vi "Event Frame Page.vi"(8 "error in (no error)":errorcluster, 11 "Node Ptr":T1 format="%.0x") -> (0 "error out":errorcluster)   [LabVIEW 2015, in "J1939 Addon System Explorer.lvlib"]
uses:
  J1939 Addon System Explorer.lvlib
  <vilib>/NI Veristand/Custom Device API/Custom Device Item Ref.ctl
  Shared/Types/XNET Frame Event Properties.ctl
  Shared/J1939 Utilities/SubVIs/Convert CAN Arb ID to J1939 ID.vi
  Shared/SubVIs/Constants.vi
  <vilib>/NI Veristand/Custom Device API/Get Item Property (U32).vi
  <vilib>/NI Veristand/Custom Device API/Get Item Property (Variant).vi
  <vilib>/NI Veristand/Custom Device API/Set Item Property (Variant).vi
  <vilib>/NI VeriStand/Custom Device API/Custom Device API.lvlib
  Shared/J1939 Addon Shared.lvlib
  Shared/J1939 Utilities/J1939 Utilities.lvlib
panel:
  in  "Description":string
  out "Source Address":u8
  out "Priority":u8
  out "PGN":u32
  in  "SHDocVw.IWebBrowser2":refnum<k7>(container)
  in  "Transimission Trigger":cluster{"Section Name":string}={"Section Name"="Transmission Trigger"}
  out "Frame ID":u32
  in  "Enable software cyclic trigger":bool
  in  "Transmit trigger":enum16{"Channel value change"}(ring)
  in  "Transmit Time":dbl format="%#_p"
  in  "Custom Device Settings":cluster{"Section Name":string}={"Section Name"="Custom Device Item Settings"}
  out "Name":string
  # "secs"
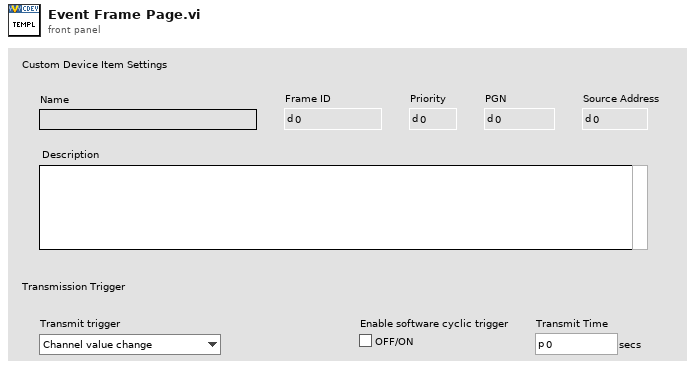
[diagram p1: front panel]
types:
  T1 = typedef "Custom Device API.lvlib/Custom Device Item Ref.ctl" = u64
  T2 = typedef "J1939 Addon Shared.lvlib/XNET Frame Event Properties.ctl" = cluster{"Transmit trigger":enum16{"Channel value change"}, "Enable software cyclic trigger":bool, "Transmit Time":dbl}
  T3 = typedef "Custom Device API.lvlib/Custom Device Item Info.ctl" = cluster{"Name":string, "Is Channel":bool, "GUID":string, "Is Waveform":bool}
  T4 = enum8{"Enabled", "Disabled", "Disabled and Grayed Out"}
  T5 = typedef "Custom Device API.lvlib/Custom Device Commands.ctl" = enum16{"Default", "Item renamed", "Shutdown", "Dynamic button pressed"}
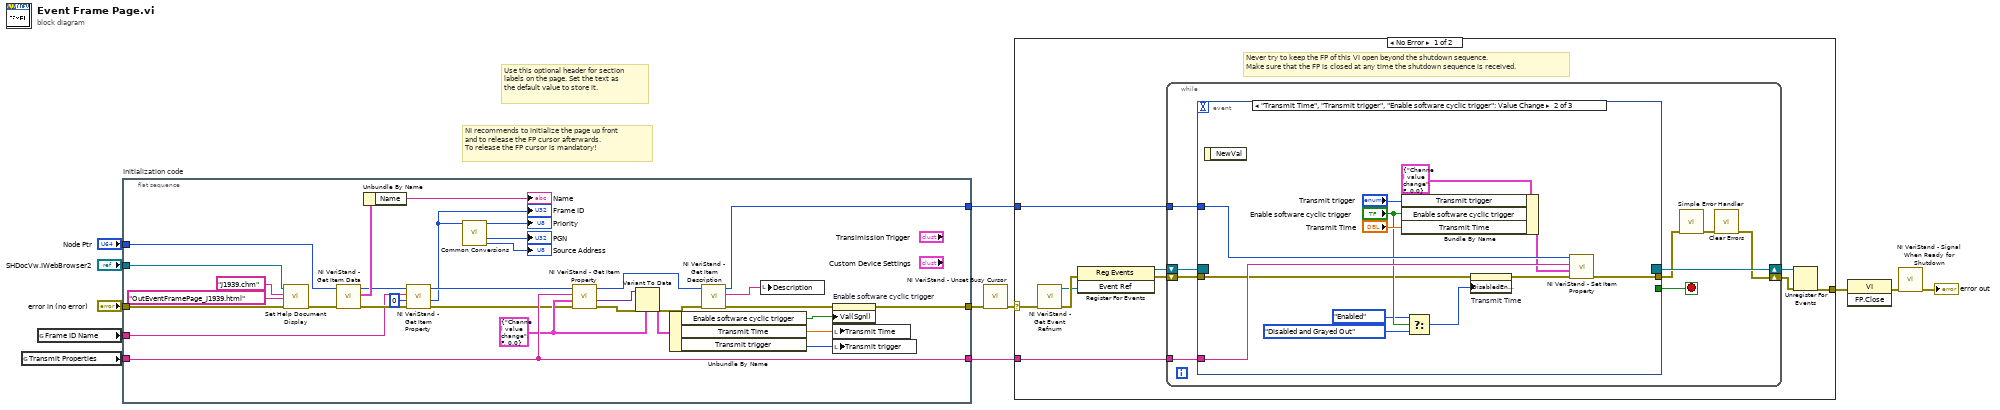
[diagram p0: block diagram]
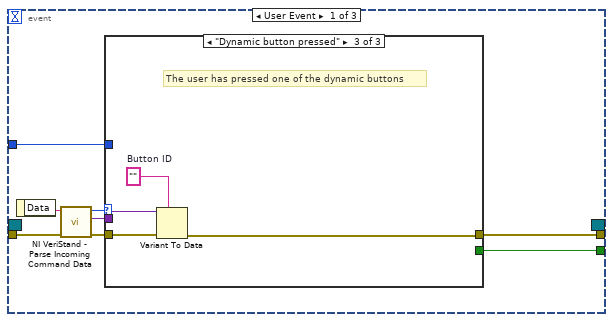
[diagram p2: hidden frame]
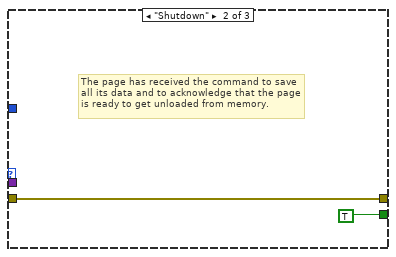
[diagram p4: hidden frame]
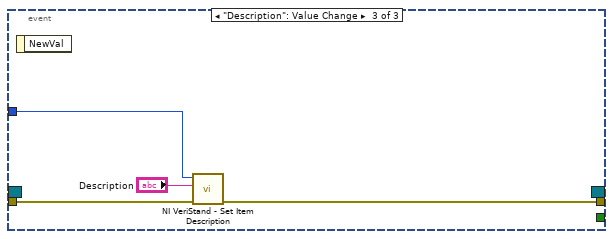
[diagram p5: hidden frame]
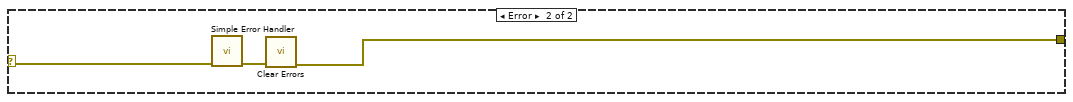
[diagram p6: hidden frame]
diagram:
  # "Use this optional header for section labels on the page. Set the text as the default value to store it."
  # "NI recommends to initialize the page up front\nand to release the FP cursor afterwards.\nTo release the FP cursor is mandatory!"
  n1 = global read "Constants.vi" "Transmit Properties"() -> (w4:string)
  n2 = global read "Constants.vi" "Frame ID Name"() -> (w1:string)
  n3 = flat-sequence "Initialization code" {
    tunnel: "error in (no error)" -> [w39]
    tunnel: "Node Ptr" -> [w42]
    tunnel: [w13] -> w8
    tunnel: [w17] -> w5
    tunnel: w4 -> [w43]
    tunnel: [w43] -> w3
    tunnel: "SHDocVw.IWebBrowser2" -> [w37]
    tunnel: w1 -> [w25]
    frame #0 {
      w34 = T2 {"Transmit trigger"=enum."Channel value change", "Enable software cyclic trigger"=FALSE, "Transmit Time"=0.0} ("Transmit Properties")
      n4 = call "Set Help Document Display.vi"("error in (no error)"=w39, "HTML File"="OutEventFramePage_J1939.html", "Main CHM File"="J1939.chm", "SHDocVw.IWebBrowser2"=w37) -> ("error out"=w38:errorcluster)  [unwired: 7 in]
      n5 = call <vilib>:"NI VeriStand - Get Item Data.vi"("error in (no error)"=w38, "Item Ref in"=w42) -> ("error out"=w30:errorcluster, "Item Info"=w44:T3, "Item Ref out"=w28:T1)  [unwired: 7 out]
      n6 = Unbundle By Name(w44) -> ("Name"=→"Name":string)
      n7 = call-poly <vilib>:"NI VeriStand - Get Item Property.vi"("error in (no error)"=w30, "Default Value"=u32 0, "Property Name"=w25, "Item Ref in"=w28) -> ("error out"=w29:errorcluster, "Value"=w24:u32, "Item Ref out"=w27:T1)  [unwired: 4 in, 1 out]
      "Frame ID" <- w24
      n8 = call-poly "Common Conversions.vi"("Arb ID"=w24) -> ("Priority"=→"Priority":u8, "PGN"=→"PGN":u32, "Source Address"=→"Source Address":u8)  [unwired: 11 in, 1 out]
      n9 = call-poly <vilib>:"NI VeriStand - Get Item Property.vi"("error in (no error)"=w29, "Default Value"=w34, "Property Name"=w43, "Item Ref in"=w27) -> ("error out"=w36:errorcluster, "Value"=w35:variant, "Item Ref out"=w18:T1)  [unwired: 4 in, 1 out]
      n10 = Variant To Data(error in=w36, type=w34, Variant=w35) -> (data=w33:T2, error out=w19:errorcluster)
      n11 = Unbundle By Name(w33) -> ("Enable software cyclic trigger"=w14:bool, "Transmit Time"=w32:dbl, "Transmit trigger"=w31:enum16{"Channel value change"})
      n12 = call <vilib>:"NI VeriStand - Get Item Description.vi"("error in (no error)"=w19, "Item Ref in"=w18) -> ("error out"=w15:errorcluster, "Description"=w16:string, "Item Ref out"=w17:T1)  [unwired: 7 out]
      n13 = local write "Description"(w16) -> ()
      n14 = property on="Enable software cyclic trigger" class="Bool (strict)"(error in=w15, "Val(Sgnl)"=w14) -> (error out=w13:errorcluster)  [unwired: 1 in, 1 out]
      n15 = local write "Transmit Time"(w32) -> ()
      n16 = local write "Transmit trigger"(w31) -> ()
    }
  }
  n17 = call <vilib>:"NI VeriStand - Unset Busy Cursor.vi"("error in (no error)"=w8) -> ("error out"=w7:errorcluster)  [unwired: 10 out]
  n18 = case shown="No Error" w7 {
    selector: w7 -> [w46 w98]
    tunnel: [w51 w96] -> w12
    tunnel: w5 -> [w47 _]
    tunnel: w3 -> [w45 _]
    frame No Error {
      # "Never try to keep the FP of this VI open beyond the shutdown sequence.\nMake sure that the FP is closed at any time the shutdown sequence is received."
      n19 = call <vilib>:"NI VeriStand - Get Event Refnum.vi"("error in (no error)"=w46) -> ("error out"=w54:errorcluster, "Event Ref"=w50:refnum<user-event>)  [unwired: 9 out]
      n20 = register-events(error in=w54, w50) -> (reference out=w48:refnum<event-registration>, error out=w49:errorcluster)  [unwired: 1 in]
      n21 = while {
        tunnel: w47 -> [w59]
        shift-right: [w56] -> w52
        shift-left: w49 -> [w62]
        shift-right: [w63] -> w53
        shift-left: w48 -> [w61]
        tunnel: w45 -> [w55]
        stop <- w60 stop-if-true
        n22 = event shown="[1] \"Transmit Time\", \"Transmit trigger\", \"Enable software cyclic trigger\": Value Change" {
          selector: w61 -> [_ _ _]
          dyn-events: [_ _ _] -> w63
          timeout: _ -> [_ _ _]
          tunnel: w62 -> [w71 w80 w94]
          tunnel: [w67 _ _] -> w60
          tunnel: [w66 w91 w93] -> w58
          tunnel: w59 -> [w65 w90 w92]
          tunnel: w55 -> [_ w89 _]
          event User Event {
            n23 = event-data() -> ("Data"=w70:string)  [unwired: 1 out]
            n24 = call <vilib>:"NI VeriStand - Parse Incoming Command Data.vi"("error in (no error)"=w71, "Incoming data"=w70) -> ("error out"=w69:errorcluster, "Outgoing data"=w64:variant, "Action"=w68:T5)  [unwired: 7 out]
            n25 = case shown="\"Dynamic button pressed\"" w68 {
              tunnel: w69 -> [w72 w73 w78]
              tunnel: [_ TRUE _] -> w67
              tunnel: [w72 w73 w75] -> w66
              tunnel: w65 -> [_ _ _]
              tunnel: w64 -> [_ _ w77]
              frame "Default", Default {
              }
              frame "Shutdown" {
                # "The page has received the command to save all its data and to acknowledge that the page is ready to get unloaded from memory."
              }
              frame "Dynamic button pressed" {
                w76 = ""  # Button ID
                # "The user has pressed one of the dynamic buttons"
                n26 = Variant To Data(error in=w78, type=w76, Variant=w77) -> (error out=w75:errorcluster)  [unwired: 1 out]
              }
            }
          }
          event "Transmit Time", "Transmit trigger", "Enable software cyclic trigger": Value Change {
            n27 = event-data() -> ()  [unwired: 2 out]
            n28 = Bundle By Name(cluster=T2 {"Transmit trigger"=enum."Channel value change", "Enable software cyclic trigger"=FALSE, "Transmit Time"=0.0} ("Transmit Properties"), "Transmit trigger"="Transmit trigger", "Enable software cyclic trigger"="Enable software cyclic trigger", "Transmit Time"="Transmit Time") -> (w85:T2)
            n29 = Select(t=T4."Enabled" ("Disabled"), s="Enable software cyclic trigger", f=T4."Disabled and Grayed Out") -> (s? t:f=w81:T4)
            n30 = property on="Transmit Time" class="DigNum (strict)"(error in=w80, "DisabledEnum"=w81) -> (error out=w79:errorcluster)  [unwired: 1 in, 1 out]
            n31 = call-poly <vilib>:"NI VeriStand - Set Item Property.vi"("error in (no error)"=w79, "Value"=w85, "Property Name"=w89, "Item Ref in"=w90) -> ("error out"=w91:errorcluster)  [unwired: 5 in, 2 out]
          }
          event "Description": Value Change {
            n32 = event-data() -> ()  [unwired: 2 out]
            n33 = call <vilib>:"NI VeriStand - Set Item Description.vi"("error in (no error)"=w94, "Description"="Description", "Item Ref in"=w92) -> ("error out"=w93:errorcluster)  [unwired: 8 out]
          }
        }
        n34 = call <vilib>:"Simple Error Handler.vi"("error in (no error)"=w58) -> ("error out"=w57:errorcluster)  [unwired: 1 in, 7 out]
        n35 = call <vilib>:"Clear Errors.vi"("error in (no error)"=w57) -> ("error out"=w56:errorcluster)  [unwired: 1 in, 5 out]
      }
      n36 = Unregister For Events(event registration refnum=w53, error in=w52) -> (error out=w51:errorcluster)
    }
    frame Error {
      n37 = call <vilib>:"Simple Error Handler.vi"("error in (no error)"=w98) -> ("error out"=w97:errorcluster)  [unwired: 1 in, 7 out]
      n38 = call <vilib>:"Clear Errors.vi"("error in (no error)"=w97) -> ("error out"=w96:errorcluster)  [unwired: 1 in, 5 out]
    }
  }
  n39 = invoke class="VI" method="FP.Close"(error in=w12) -> (error out=w11:errorcluster)  [unwired: 2 in, 2 out]
  n40 = call <vilib>:"NI VeriStand - Signal When Ready for Shutdown.vi"("error in (no error)"=w11) -> ("error out"=→"error out":errorcluster)  [unwired: 10 out]
